vi "CE XCL Write measurement line.vi"(6 "Iteration index":i32, 7 "report in":refnum<class "NI_report.lvclass">, 8 "error in (no error)":errorcluster, 9 "TWM result as string for XCL":string[][](array[string]), 11 "CE measurement":T1={"Signal frequencies (Hz) T"=[1000.0], "Signal amplitudes (V) T"=[0.707], "Sampling frequencies (Hz) T"=[10000000.0], "Record lengths (multiples of periods) T"=[10000.0], "TWM data root directory"=path "", "TWM mreasurements directories"=[], "Calculate RMS from samples"=FALSE, "Algorithm to use"="TWM-WFFT", "Quantity to read"="TWM-WFFT", "Settle down after AC source change (s) T"=1.0, "Skip PJVS setup"=FALSE, "Measurement template file"=path "", "Row of START keyword T"=0, "Row of STOP keyword T"=0, "Measurement template line T"=[], "Switch position T"=[10000.0], "FR fit mat file T"=path "", "Recalculate-skip already calculated"=FALSE} {"Switch position T" format="%#_3p"; "Record lengths (multiples of periods) T" format="%#_3p"; "Sampling frequencies (Hz) T" format="%#_3p"; "Signal amplitudes (V) T" format="%#_3p"; "Signal frequencies (Hz) T" format="%#_3p"}) -> (0 "error out":errorcluster, 5 "report out":refnum<class "NI_report.lvclass">)   [LabVIEW 2020]
doc: "Writes measurement results for a single line in CE template."
uses:
  <vilib>/Utility/NIReport.llb/NI_report.lvclass
  CE Measurement/Type definitions/CE measurement.ctl
  external libraries/varilib/varilib.lvlib
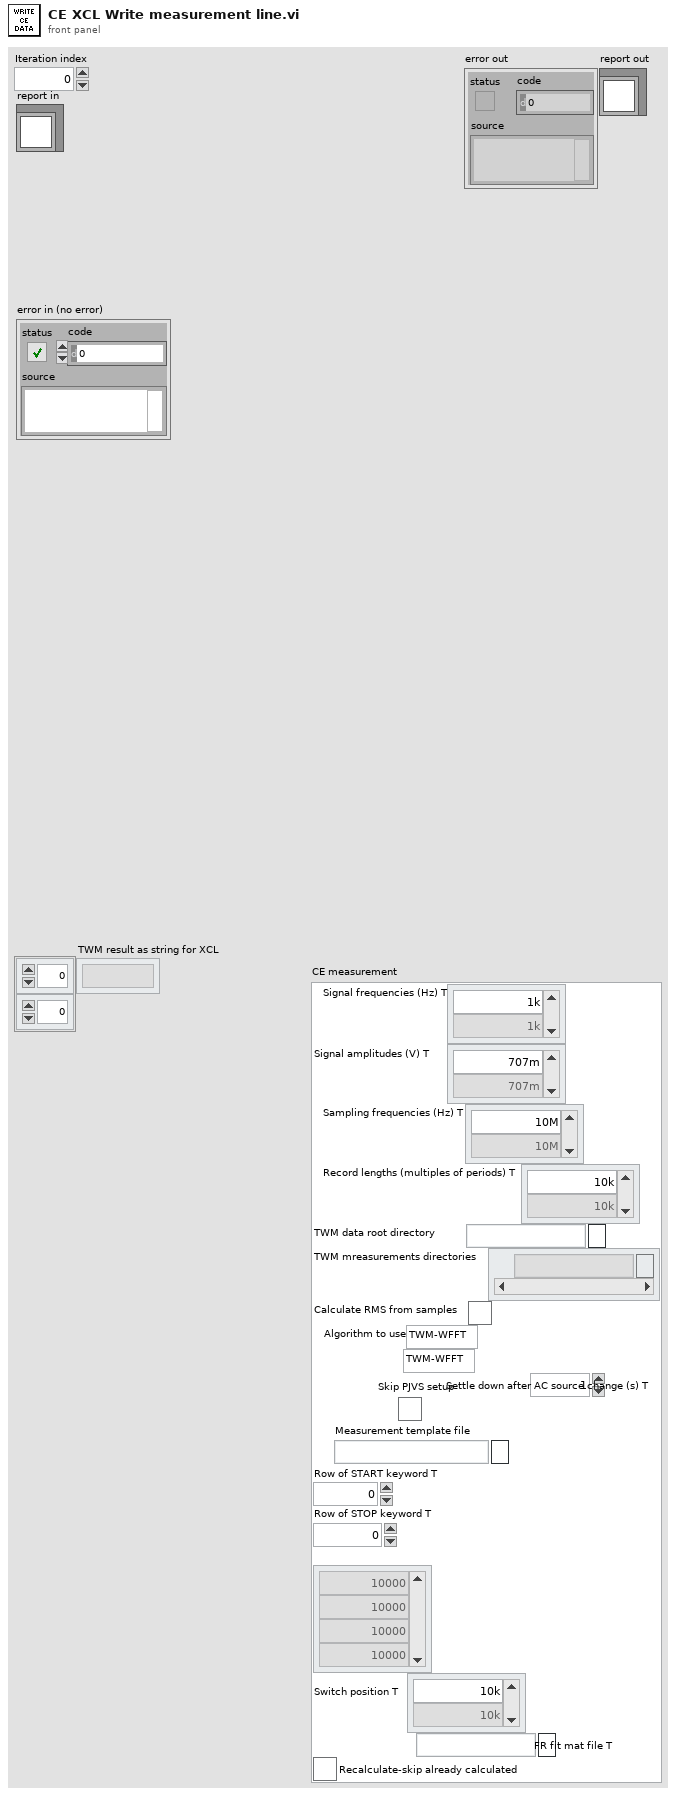
[diagram p1: front panel]
types:
  T1 = typedef "CE measurement.ctl" = cluster{"Signal frequencies (Hz) T":dbl[], "Signal amplitudes (V) T":dbl[], "Sampling frequencies (Hz) T":dbl[], "Record lengths (multiples of periods) T":dbl[], "TWM data root directory":path, "TWM mreasurements directories":path[], "Calculate RMS from samples":bool, "Algorithm to use":string, "Quantity to read":string, "Settle down after AC source change (s) T":dbl, "Skip PJVS setup":bool, "Measurement template file":path, "Row of START keyword T":i32, "Row of STOP keyword T":i32, "Measurement template line T":i32[], "Switch position T":dbl[], "FR fit mat file T":path, "Recalculate-skip already calculated":bool}
  T2 = typedef "Type definitions to be saved.ctl" = cluster{"Common properties":T3, "AC Source":T4, "DC meter":T6, "CE measurement":T1, "FR measurement":T8, "FR template":T9, "CE template":T10, "PJVS":T11, "SS measurement":T15, "AC sync source":T4, "DG measurement":T16}
  T3 = typedef "Common properties.ctl" = cluster{"Measurement status ref":refnum<vi>, "TWM Status ref":refnum<vi>, "Abort ref":refnum<vi>, "Skip waiting ref":refnum<vi>, "GNU Octave path":path, "TWM+QWTB path":path, "lvlib path":path, "TWM pipe":string, "PJVS status ref":refnum<vi>, "WAC path":path}
  T4 = typedef "AC Source.ctl" = cluster{"AC Source type":T5, "VISA":refnum<visa-resource-name>, "Ref. clock (Hz)":dbl, "status ref":refnum<vi>, "Fluke 57XX wideband output":bool, "Fluke 57XX ignore errors":bool, "Synchronization by AC signal":bool}
  T5 = typedef "AC Source type.ctl" = enum16{"Fluke 5XXX calibrator", "Tektronix AFG3000 series", "dummy", "Agilent 331xxA to 332xxA", "Agilent 335xxA to 336xxA"}
  T6 = typedef "DC meter.ctl" = cluster{"DC meter type":T7, "DC meter VISA":refnum<visa-resource-name>, "NPLC":dbl, "status ref":refnum<vi>}
  T7 = typedef "DC meter type.ctl" = enum16{"H/A/K 3458", "Fluke 8508A", "dummy", "Keithley 2182"}
  T8 = typedef "FR measuement.ctl" = cluster{"Measurement frequencies (Hz)":dbl[], "Sampling frequency (Hz)":dbl, "Signal amplitude (V)":dbl, "AC-DC settle time (s)":dbl, "Record length (multiples of period)":dbl[], "Measurement template file":path, "Row of START keyword":i32, "Row of STOP keyword":i32, "Calculate RMS from samples":bool, "AC-DC warm up time (s)":dbl, "Measurement template line":i32[], "DC meter readings No.":i32, "Algorithm":string, "Simultaneous measurement":bool, "Recalculate-skip already calculated":bool}
  T9 = typedef "FR template.ctl" = cluster{"Keywords column":i32, "Sig. freq. column":i32, "Rec. len. column":i32, "Meas. points. row min to read":i32, "Meas. points. row max to read":i32, "Properties column":i32, "Properties row start":i32, "Properties row end":i32, "Keyword START regexp":string, "Keyword STOP regexp":string, "HW data column":i32, "HW data row start":i32, "HW data row end":i32, "TIme and date column start":i32, "Digitizer value column start ":i32, "DC mean column start ":i32, "DC readings column start":i32}
  T10 = typedef "CE template.ctl" = cluster{"Keywords column":i32, "Sig. freq. column":i32, "Rec. len. column":i32, "Switch pos column":i32, "Meas. points. row min to read":i32, "Meas. points. row max to read":i32, "Properties column":i32, "Properties row start":i32, "Properties row end":i32, "Keyword START regexp":string, "Keyword STOP regexp":string, "HW data column":i32, "HW data row start":i32, "HW data row end":i32, "TIme and date column start":i32, "Digitizer value column start ":i32}
  T11 = typedef "PJVS.ctl" = cluster{"PJVS type":T12, "Status Refnum":refnum<vi>, "AC-supraVOLTcontrol":cluster{"IP address:port (0.0.0.0:0000)":string, "Timeouts":T13, "Simulation mode":bool, "Debug mode":bool}, "NPL bias source":cluster{"DataSocketCluster":T14}, "Manual PJVS":cluster{"PJVS frequency (Hz)":dbl, "Reference voltages (V)":dbl[], "File with PJVS voltages":path}, "VTT PJVS":cluster{"some VTT only property":string}}
  T12 = typedef "PJVS Type.ctl" = enum16{"AC-supraVOLTcontrol", "JV modified NPL bias control", "Manual PJVS", "VTT PJVS"}
  T13 = typedef "ACSVcontrol-driver.lvlib/Timeouts.ctl" = cluster{"TCP Read & Write (ms)":i32, "Sensors readout":i32, "PJVS setup":i32, "Nullmeter readout":i32, "Multiplexer setup":i32, "57XX setup":i32, "Generator setup":i32, "Synthesizer setup":i32, "Sampler readout":i32}
  T14 = typedef "DataSocketCluster external.ctl" = cluster{"Server Machine":string, "Client Machine":string, "Data":string, "TimeStamp":dbl, "Count":i32, "Target Process":string}
  T15 = typedef "SS measurement.ctl" = cluster{"Signal frequencies (Hz)":dbl[], "Signal amplitudes (V)":dbl[], "Sampling frequencies (Hz)":dbl[], "Record lengths (multiples of periods)":dbl[], "Calculate results":bool, "Algorithm":string, "TWM data directories":path[], "TWM data directories relative":path[], "Settle down after AC source change (s)":dbl, "PJVS frequencies (Hz)":dbl[], "PJVS reference voltages array of vector cluster":cluster{"PJVS reference voltages vector":dbl[]}[], "Requested PJVS steps":u32[], "Measure CE":bool, "Measure CE before":bool, "Measure CE after":bool, "Single point CE measurement":bool, "original CE template path":path, "new CE template path before SS":path, "new CE template path before SS relative":path, "new CE template path after SS":path, "new CE template path after SS relative":path, "original CE fit path":path, "new CE fit path before SS":path, "new CE fit path before SS relative":path, "new CE fit path after SS":path, "new CE fit path after SS relative":path, "Measure digitizer gain":bool, "Measure digitizer gain before":bool, "Measure digitizer gain after":bool, "Digitizer gain":dbl, "Data folder":path, "FR fit path":path, "new FR fit path relative":path, "Rs":i32, "Re":i32, "SS measurement info files":path[]}
  T16 = typedef "DG measurement.ctl" = cluster{"Sampling frequencies (Hz)":dbl[], "Requested PJVS frequencies (Hz)":dbl[], "Requested PJVS waveform amplitudes (V)":dbl[], "Record lengths (multiples of PJVS periods)":dbl[], "Requested PJVS steps":u32[], "Switch position":dbl, "Settle down after PJVS change (s)":dbl, "Rs":i32, "Re":i32, "Algorithm":string, "Calculate results":bool, "Data folder":path, "TWM data directories":path[], "TWM data directories relative":path[], "DG measurement info files":path[], "Set PJVS frequencies (Hz)":dbl[], "Set PJVS reference voltages array of vector cluster":cluster{"PJVS reference voltages vector":dbl[]}[], "Set PJVS steps":u32[]}
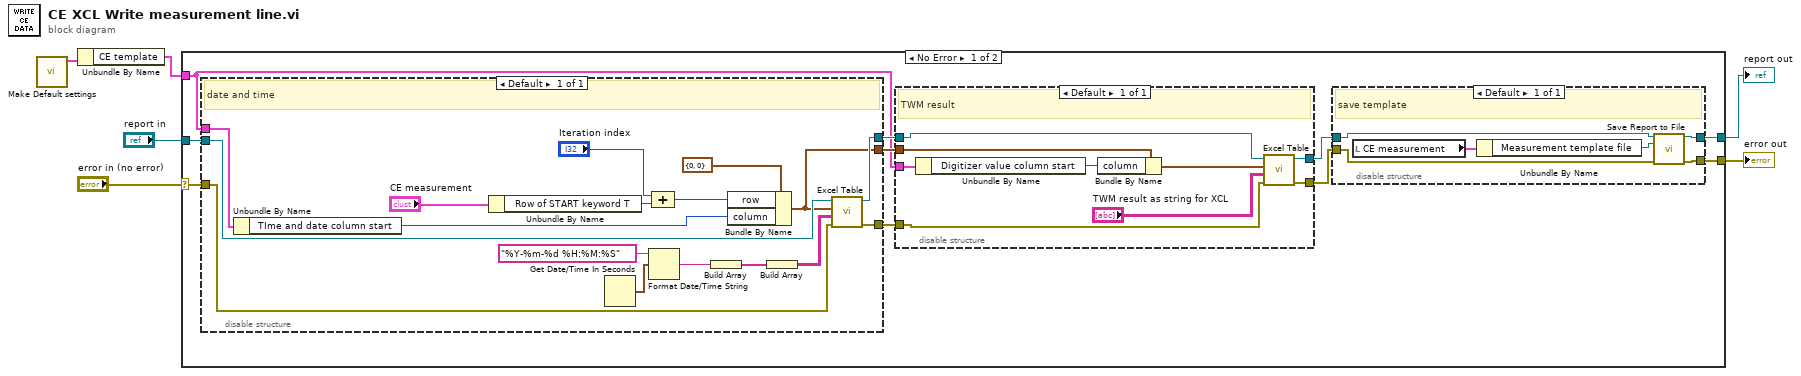
[diagram p0: block diagram]
diagram:
  n1 = call "Make Default settings.vi"() -> ("TD to be saved"=w2:T2)  [unwired: 11 in]
  n2 = Unbundle By Name(w2) -> ("CE template"=w1:T10)
  n3 = case shown="No Error" "error in (no error)" {
    selector: "error in (no error)" -> [w16 w50]
    tunnel: [w14 w50] -> w6
    tunnel: "report in" -> [w15 w49]
    tunnel: [w13 w49] -> w3
    tunnel: w1 -> [w7 _]
    frame No Error {
      n4 = disable-structure shown="Default" {
        disable-tunnel: w16 -> [w43]
        disable-tunnel: w15 -> [w42]
        disable-tunnel: [w41] -> w9
        disable-tunnel: [w40] -> w10
        disable-tunnel: [w39] -> w8
        disable-tunnel: w7 -> [w33]
        frame Enabled {
          # "date and time"
          n5 = Unbundle By Name(w33) -> ("TIme and date column start"=w32:i32)
          n6 = Unbundle By Name("CE measurement") -> ("Row of START keyword T"=w35:i32)
          n7 = Get Date/Time In Seconds() -> (seconds since 1Jan1904=w44:timestamp)
          n8 = Format Date/Time String(time format string (%c)="%Y-%m-%d %H:%M:%S", seconds (now)=w44) -> (date/time string=w46:string)  [unwired: 1 in]
          n9 = Compound Arithmetic op=ADD("Iteration index", w35) -> (w38:i32)
          n10 = Build Array(w46) -> (w47:string[])
          n11 = Bundle By Name(cluster=cluster{"row":i32, "column":i32} {"row"=0, "column"=0} ("start (0, 0)"), "row"=w38, "column"=w32) -> (w39:cluster{"row":i32, "column":i32})
          n12 = Build Array(w47) -> (w48:string[][])
          n13 = call "Excel Table.vi"("error in (no error)"=w43, "table"=w48, "start (0, 0)"=w39, "report in"=w42) -> ("error out"=w41:errorcluster, "report out"=w40:refnum<class "NI_report.lvclass">)  [unwired: 6 in]
        }
      }
      n14 = disable-structure shown="Default" {
        disable-tunnel: w9 -> [w31]
        disable-tunnel: w10 -> [w30]
        disable-tunnel: [w29] -> w12
        disable-tunnel: [w28] -> w11
        disable-tunnel: w8 -> [w27]
        disable-tunnel: w7 -> [w24]
        frame Enabled {
          # "TWM result"
          n15 = Unbundle By Name(w24) -> ("Digitizer value column start"=w23:i32)
          n16 = Bundle By Name(cluster=w27, "column"=w23) -> (w26:cluster{"row":i32, "column":i32})
          n17 = call "Excel Table.vi"("error in (no error)"=w31, "table"="TWM result as string for XCL", "start (0, 0)"=w26, "report in"=w30) -> ("error out"=w29:errorcluster, "report out"=w28:refnum<class "NI_report.lvclass">)  [unwired: 6 in]
        }
      }
      n18 = disable-structure shown="Default" {
        disable-tunnel: [w22] -> w14
        disable-tunnel: [w21] -> w13
        disable-tunnel: w12 -> [w20]
        disable-tunnel: w11 -> [w19]
        frame Enabled {
          # "save template"
          n19 = local read "CE measurement"() -> (w18:T1)
          n20 = Unbundle By Name(w18) -> ("Measurement template file"=w17:path)
          n21 = call-dynamic "Save Report to File.vi"("report in"=w19, "report file path"=w17, "error in (no error)"=w20) -> ("report out"=w21:refnum<class "NI_report.lvclass">, "error out"=w22:errorcluster)  [unwired: 11 in]
        }
      }
    }
    frame Error {
    }
  }
  "error out" <- w6
  "report out" <- w3
